vi "骰子賭聖.vi"() -> ()   [LabVIEW 2014]
panel:
  in  "Listbox 3":i32[](listbox)
  in  "Listbox 2":i32[](listbox)
  in  "Listbox":i32[](listbox)
  in  "遊戲開始":bool
  out "賭金金額":i32
  in  "Cluster":T1
  in  "結束遊戲":bool
  # "遊戲介紹:"
  # "遊戲操作:"
  # "注意事項:"
  # "看完以上說明沒問題的話，就\n點擊遊戲開始來開始賭聖之路吧!\n                       ↓"
  # "介紹:玩家對即將\n擲出的骰子的各\n類型組合進行下注"
  # "介紹:和電腦莊家\n分別擲一顆骰子\n比點數大小"
  # "介紹:用十八仔規\n則和電腦莊家分\n別擲骰子比點數\n大小"
  # "賠率:1、3、5\n下注金額:10~50"
  # "賠率:1~5\n下注金額:10~30"
  # "賠率:3~8\n下注金額:10~30"
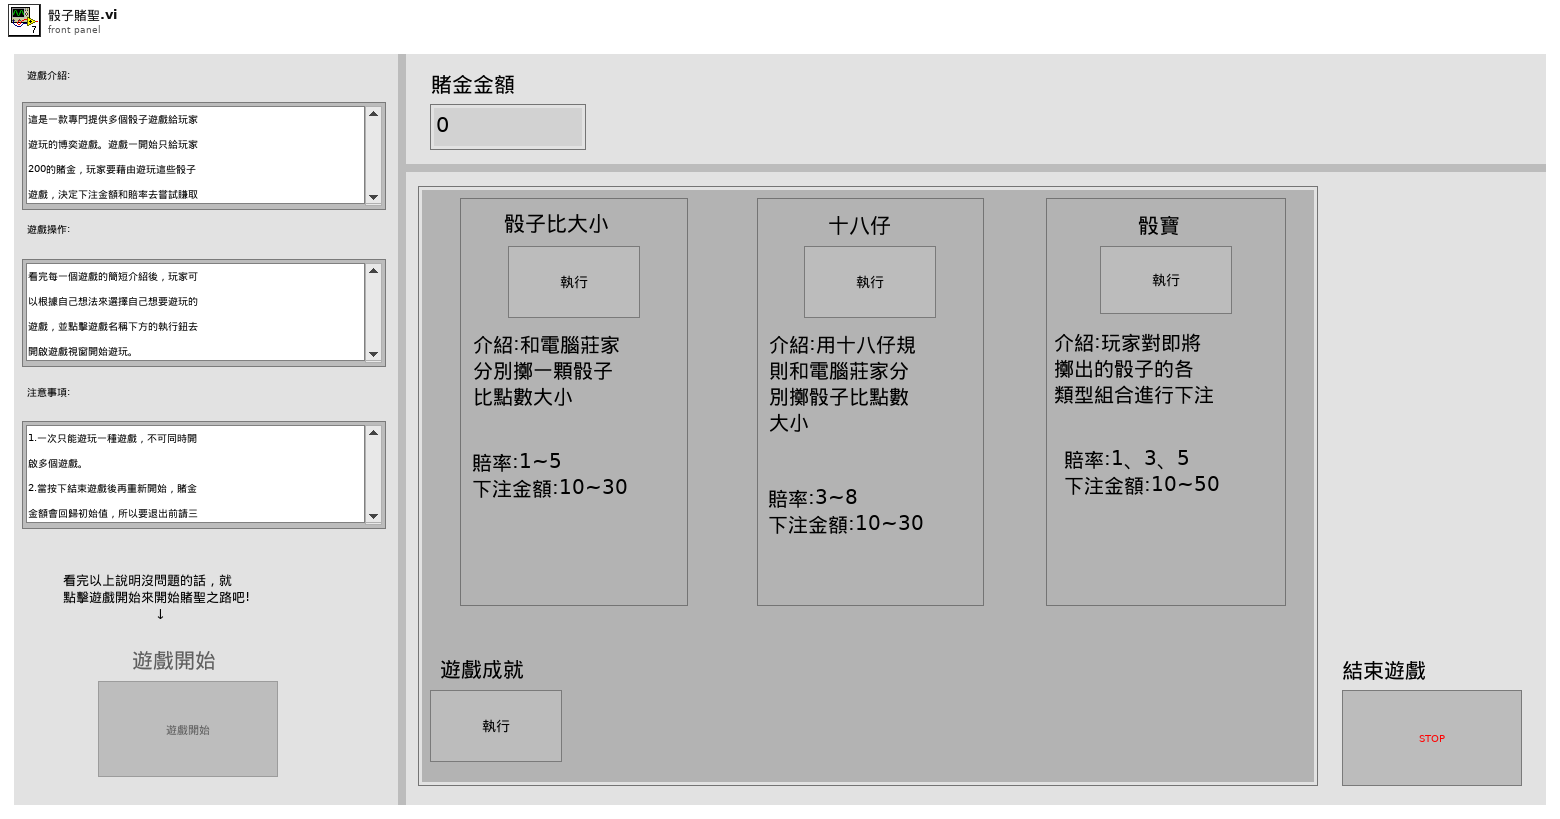
[diagram p1: front panel]
types:
  T1 = cluster{"骰子比大小":bool, "十八仔":bool, "骰寶":bool, "遊戲成就":bool}
  T2 = enum16{"money  return  ", "title", "game3", "game2", "game1", "select item", "wait start button press", "init"}
  T3 = enum8{"Enabled", "Disabled", "Disabled and Grayed Out"}
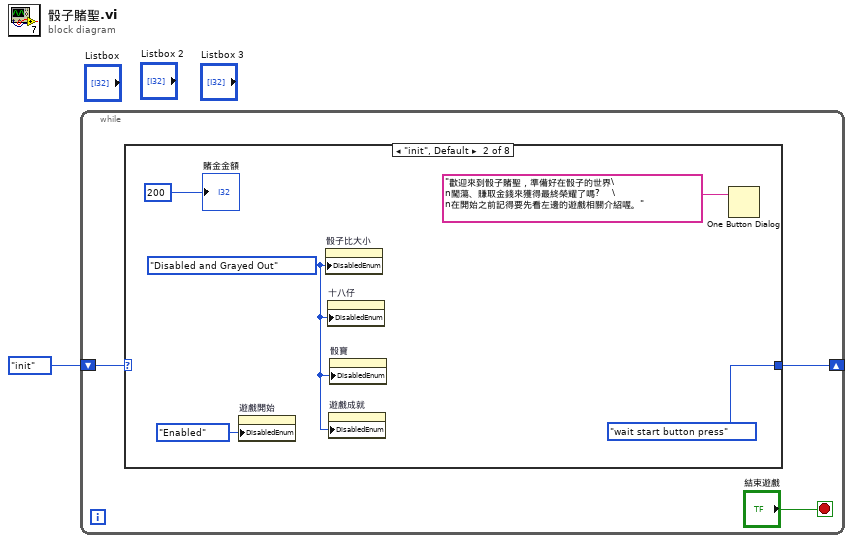
[diagram p0: block diagram]
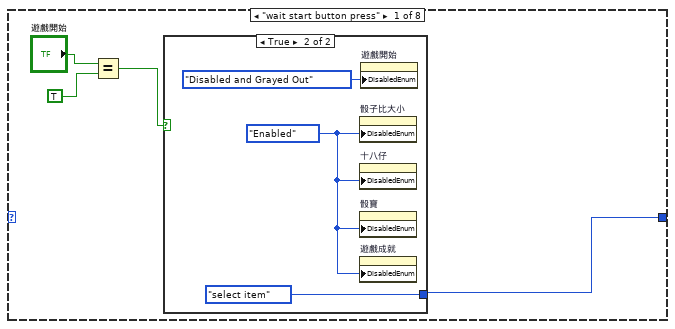
[diagram p2: hidden frame]
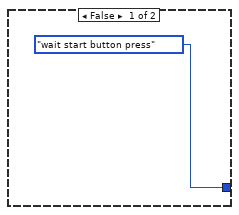
[diagram p3: hidden frame]
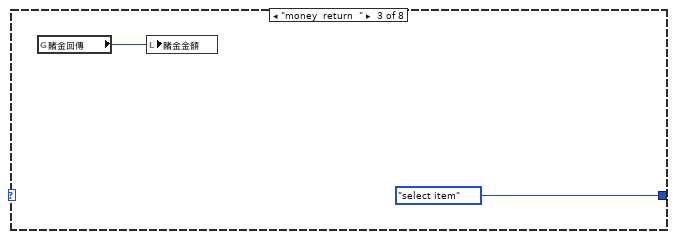
[diagram p4: hidden frame]
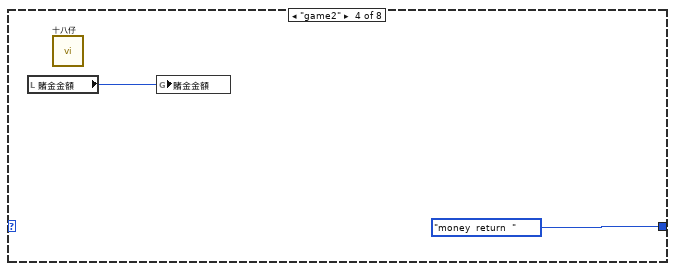
[diagram p5: hidden frame]
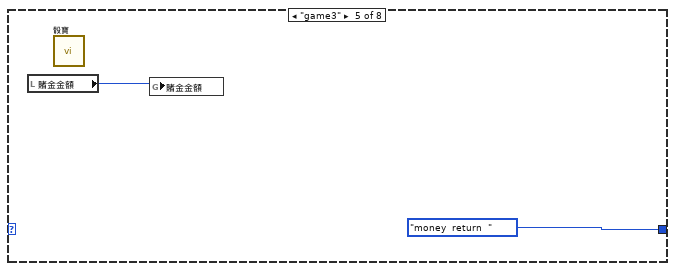
[diagram p6: hidden frame]
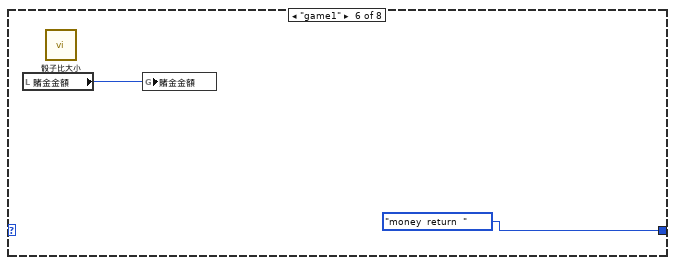
[diagram p7: hidden frame]
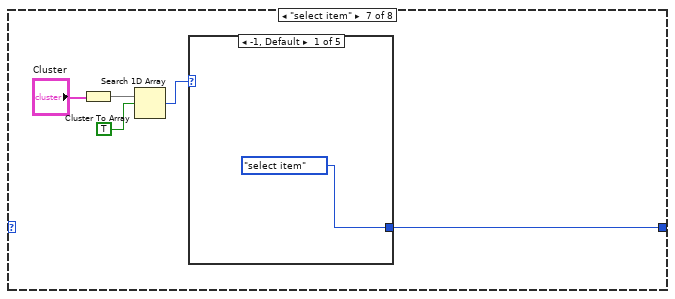
[diagram p8: hidden frame]
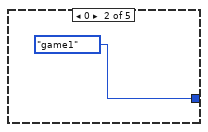
[diagram p9: hidden frame]
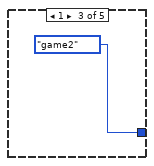
[diagram p10: hidden frame]
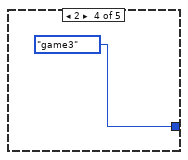
[diagram p11: hidden frame]
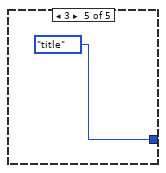
[diagram p12: hidden frame]
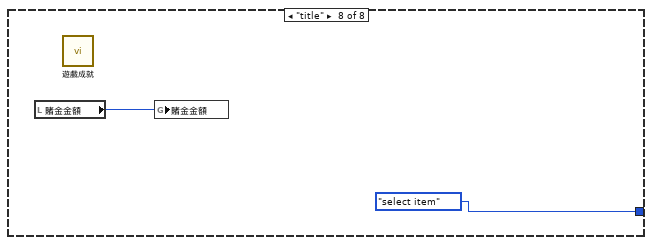
[diagram p13: hidden frame]
diagram:
  n1 = while {
    shift-right: [w2] -> _
    shift-left: T2."init" -> [w3]
    stop <- "結束遊戲" stop-if-true
    n2 = case shown="\"init\", Default" w3 {
      tunnel: [w5 T2."wait start button press" T2."select item" T2."money  return  " T2."money  return  " T2."money  return  " w26 T2."select item"] -> w2
      frame "wait start button press" {
        n3 = Equal?(x="遊戲開始", y=TRUE) -> (x = y?=w6:bool)
        n4 = case shown="True" w6 {
          tunnel: [T2."wait start button press" T2."select item"] -> w5
          frame False {
          }
          frame True {
            w10 = T3."Enabled" ("Disabled")
            n5 = property on="骰子比大小" class="Bool"("DisabledEnum"=w10) -> ()  [unwired: 2 in, 2 out]
            n6 = property on="十八仔" class="Bool"("DisabledEnum"=w10) -> ()  [unwired: 2 in, 2 out]
            n7 = property on="骰寶" class="Bool"("DisabledEnum"=w10) -> ()  [unwired: 2 in, 2 out]
            n8 = property on="遊戲成就" class="Bool"("DisabledEnum"=w10) -> ()  [unwired: 2 in, 2 out]
            n9 = property on="遊戲開始" class="Bool"("DisabledEnum"=T3."Disabled and Grayed Out" ("Disabled")) -> ()  [unwired: 2 in, 2 out]
          }
        }
      }
      frame "init", Default {
        w14 = T3."Disabled and Grayed Out" ("Disabled")
        n10 = property on="遊戲開始" class="Bool"("DisabledEnum"=T3."Enabled" ("Disabled")) -> ()  [unwired: 2 in, 2 out]
        n11 = property on="骰子比大小" class="Bool"("DisabledEnum"=w14) -> ()  [unwired: 2 in, 2 out]
        n12 = property on="十八仔" class="Bool"("DisabledEnum"=w14) -> ()  [unwired: 2 in, 2 out]
        n13 = property on="遊戲成就" class="Bool"("DisabledEnum"=w14) -> ()  [unwired: 2 in, 2 out]
        n14 = property on="骰寶" class="Bool"("DisabledEnum"=w14) -> ()  [unwired: 2 in, 2 out]
        n15 = One Button Dialog(message="歡迎來到骰子賭聖，準備好在骰子的世界\n闖蕩、賺取金錢來獲得最終榮耀了嗎?    \n在開始之前記得要先看左邊的遊戲相關介紹喔。") -> ()  [unwired: 1 in, 1 out]
        "賭金金額" <- 200
      }
      frame "money  return  " {
        n16 = global read "global variable-賭金回傳.vi" "賭金回傳"() -> (w19:i32)
        n17 = local write "賭金金額"(w19) -> ()
      }
      frame "game2" {
        n18 = local read "賭金金額"() -> (w21:i32)
        n19 = call "十八仔.vi"() -> ()  [unwired: 12 in]
        n20 = global write "global variable-賭金金額.vi" "賭金金額"(w21) -> ()
      }
      frame "game3" {
        n21 = local read "賭金金額"() -> (w23:i32)
        n22 = call "骰寶.vi"() -> ()  [unwired: 12 in]
        n23 = global write "global variable-賭金金額.vi" "賭金金額"(w23) -> ()
      }
      frame "game1" {
        n24 = local read "賭金金額"() -> (w25:i32)
        n25 = call "骰子比大小.vi"() -> ()  [unwired: 12 in]
        n26 = global write "global variable-賭金金額.vi" "賭金金額"(w25) -> ()
      }
      frame "select item" {
        n27 = Cluster To Array(cluster="Cluster") -> (array=w29:bool[])
        n28 = Search 1D Array(1D array=w29, element=TRUE) -> (index of element=w27:i32)  [unwired: 1 in]
        n29 = case shown="-1, Default" w27 {
          tunnel: [T2."select item" T2."game1" T2."game2" T2."game3" T2."title"] -> w26
          frame -1, Default {
          }
          frame 0 {
          }
          frame 1 {
          }
          frame 2 {
          }
          frame 3 {
          }
        }
      }
      frame "title" {
        n30 = local read "賭金金額"() -> (w36:i32)
        n31 = call "遊戲成就.vi"() -> ()  [unwired: 12 in]
        n32 = global write "global variable-賭金金額.vi" "賭金金額"(w36) -> ()
      }
    }
  }
